vi "Read Page Button Properties.vi"(8 "Error In":errorcluster, 11 "Custom Device Page .NET Ref In":refnum<k24>) -> (0 "Error Out":errorcluster, 2 "All Button Properties":T1[](array[typedef]), 3 "Custom Device Page .NET Ref Out":refnum<k24>)   [LabVIEW 2015, in "VeriStand XML Parser.lvlib"]
doc: "Reads and returns the properties of all buttons for the page"
uses:
  VeriStand XML Parser.lvlib
  XML Controls/Button Properties.ctl
  XML Controls/Path Cluster.ctl
  XML Controls/Button Type.ctl
  XML Controls/Dependency Properties.ctl
  NationalInstruments.VeriStand.XMLReader
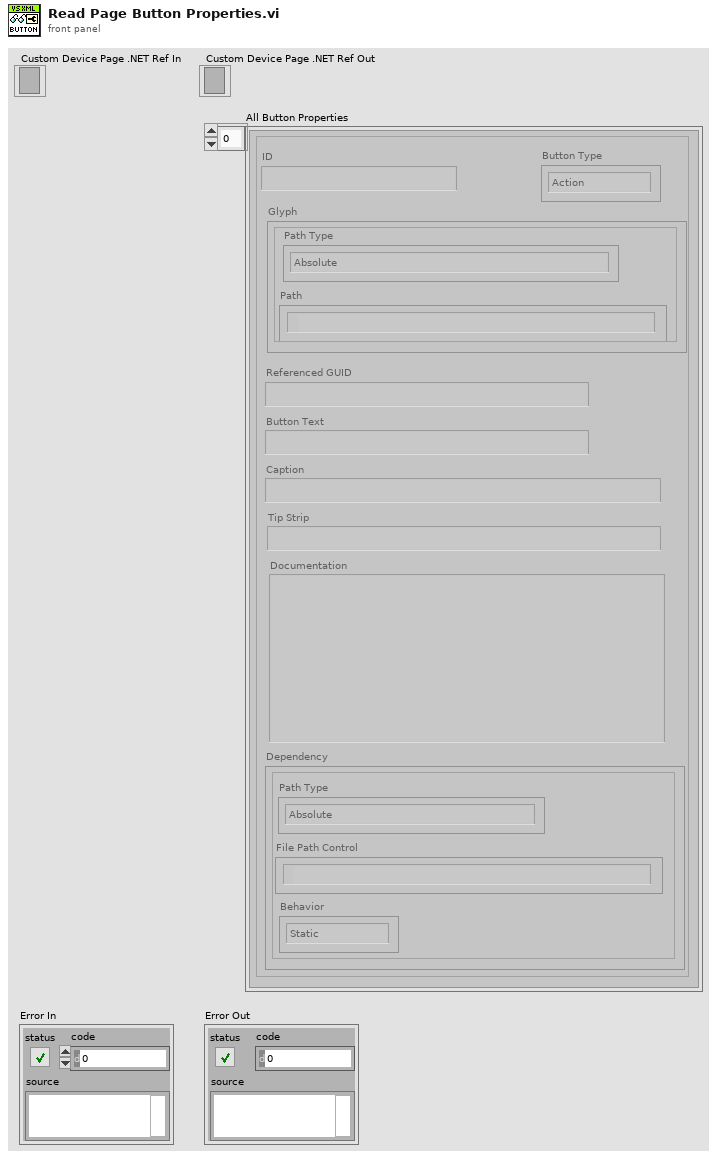
[diagram p1: front panel]
types:
  T1 = typedef "VeriStand XML Parser.lvlib/Button Properties.ctl" = cluster{"ID":string, "Glyph":T2, "Button Type":T3, "Referenced GUID":string, "Button Text":string, "Caption":string, "Tip Strip":string, "Documentation":string, "Dependency":T4}
  T2 = typedef "VeriStand XML Parser.lvlib/Path Cluster.ctl" = cluster{"Path":path, "Path Type":enum16{"Absolute", "To Base", "To Common Doc Dir", "To Application Data Dir"}}
  T3 = typedef "VeriStand XML Parser.lvlib/Button Type.ctl" = enum16{"Action", "Dialog", "Page", "Notification", "Separator"}
  T4 = typedef "VeriStand XML Parser.lvlib/Dependency Properties.ctl" = cluster{"File Path Control":path, "Path Type":enum16{"Absolute", "To Base", "To Common Doc Dir", "To Application Data Dir"}, "Behavior":enum16{"Static", "Dynamic"}}
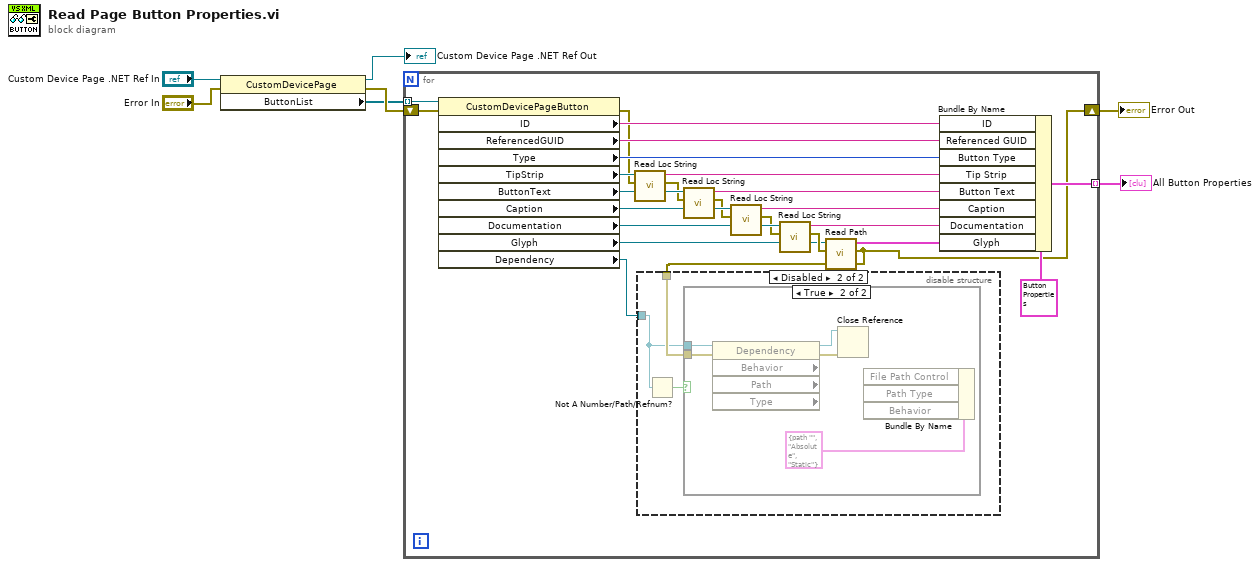
[diagram p0: block diagram]
diagram:
  n1 = property class="CustomDevicePage"(reference="Custom Device Page .NET Ref In", error in="Error In") -> (reference out=→"Custom Device Page .NET Ref Out":refnum<k24>, error out=w4:errorcluster, "ButtonList"=w3:refnum<k24>[])
  n2 = for {
    tunnel: w3 -> [w30] mode=indexing
    shift-right: [w8] -> w6
    shift-left: w4 -> [w31]
    tunnel: [w9] -> w7 mode=indexing
    n3 = property class="CustomDevicePageButton"(reference=w30, error in=w31) -> (error out=w24:errorcluster, "ID"=w28:string, "ReferencedGUID"=w27:string, "Type"=w26:i32, "TipStrip"=w25:refnum<k24>, "ButtonText"=w22:refnum<k24>, "Caption"=w19:refnum<k24>, "Documentation"=w18:refnum<k24>, "Glyph"=w14:refnum<k24>, "Dependency"=w10:refnum<k24>)  [unwired: 1 out]
    n4 = call "Read Loc String.vi"("Error In"=w24, "Loc String .NET Ref"=w25) -> ("Error Out"=w21:errorcluster, "English"=w23:string)  [unwired: 7 in, 1 out]
    n5 = call "Read Loc String.vi"("Error In"=w21, "Loc String .NET Ref"=w22) -> ("Error Out"=w17:errorcluster, "English"=w20:string)  [unwired: 7 in, 1 out]
    n6 = call "Read Loc String.vi"("Error In"=w17, "Loc String .NET Ref"=w19) -> ("Error Out"=w16:errorcluster, "English"=w13:string)  [unwired: 7 in, 1 out]
    n7 = call "Read Loc String.vi"("Error In"=w16, "Loc String .NET Ref"=w18) -> ("Error Out"=w15:errorcluster, "English"=w12:string)  [unwired: 7 in, 1 out]
    n8 = call "Read Path.vi"("Error In"=w15, "Path .NET Ref"=w14) -> ("Error Out"=w8:errorcluster, "Path Properties"=w11:T2)  [unwired: 8 in]
    n9 = disable-structure shown="Disabled" {
      disable-tunnel: w10 -> [_ w32]
      disable-tunnel: w8 -> [_ w33]
      frame Enabled {
        # "#Bug - Don't properly handle dependency. Need\nfront end changes to get all necessary data"
      }
      frame Disabled {
        n10 = Not A Number/Path/Refnum?(number/path/refnum=w32) -> (NaN/Path/Refnum?=w34:bool)
        n11 = case shown="True" w34 {
          tunnel: w33 -> [_ w39]
          tunnel: w32 -> [_ w38]
          frame False {
          }
          frame True {
            n12 = property class="Dependency" props=["Behavior", "Path", "Type"](reference=w38, error in=w39) -> (reference out=w36:refnum<k24>, error out=w37:errorcluster)  [unwired: 3 out]
            n13 = Close Reference(reference=w36, error in (no error)=w37) -> ()  [unwired: 1 out]
            n14 = Bundle By Name(cluster=T4 {"File Path Control"=path "", "Path Type"=enum."Absolute", "Behavior"=enum."Static"} ("Dependency")) -> ()  [unwired: 3 in, 1 out]
          }
        }
      }
    }
    n15 = Bundle By Name(cluster=T1 {"ID"="", "Glyph"={"Path"=path "", "Path Type"=enum."Absolute"}, "Button Type"=enum."Action", "Referenced GUID"="", "Button Text"="", "Caption"="", "Tip Strip"="", "Documentation"="", "Dependency"={"File Path Control"=path "", "Path Type"=enum."Absolute", "Behavior"=enum."Static"}} ("Button"), "ID"=w28, "Referenced GUID"=w27, "Button Type"=w26, "Tip Strip"=w23, "Button Text"=w20, "Caption"=w13, "Documentation"=w12, "Glyph"=w11) -> (w9:T1)
  }
  "All Button Properties" <- w7
  "Error Out" <- w6
